vi "Microscope Controller GFV.vi"(8 "error in (no error)":errorcluster, 10 "MicroscopeEnum":T1, 11 "Data in":variant) -> (0 "error out":errorcluster, 3 "Data Out":variant)   [LabVIEW 2017]
doc: "Use this template to build a VI to use as a subVI."
uses:
  Microscope/MicroscopeControllerEnum.ctl
  Microscope/MicroscopeControllerCluster.ctl
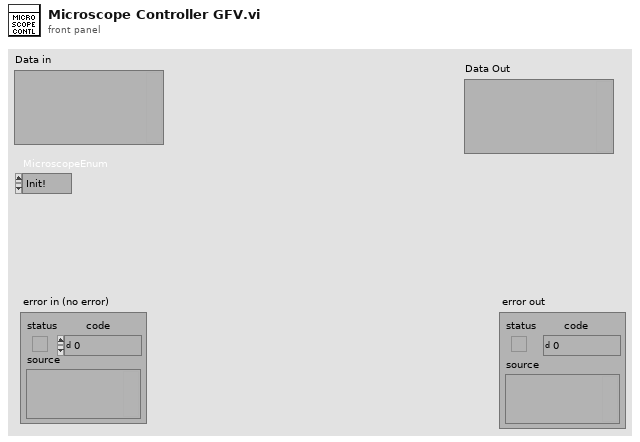
[diagram p1: front panel]
types:
  T1 = typedef "MicroscopeControllerEnum.ctl" = enum16{"Init!", "Start!", "Stop!", "GetMicroscopeVIRef", "InsertCallbackEvent!"}
  T2 = typedef "MicroscopeControllerCluster.ctl" = cluster{"MapPointsArray":cluster{"X":i32, "Y":i32}[], "Laser Point Coor":cluster{"X":i32, "Y":i32}, "Microscope \nObjective":u16}
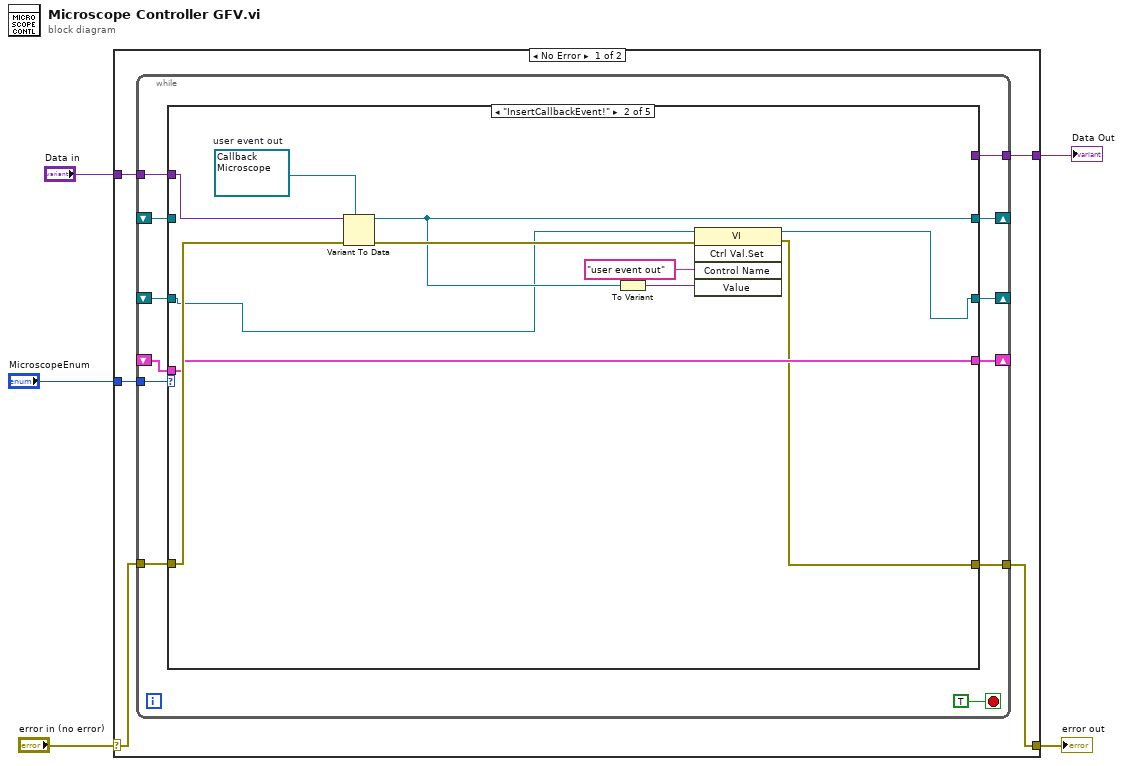
[diagram p0: block diagram]
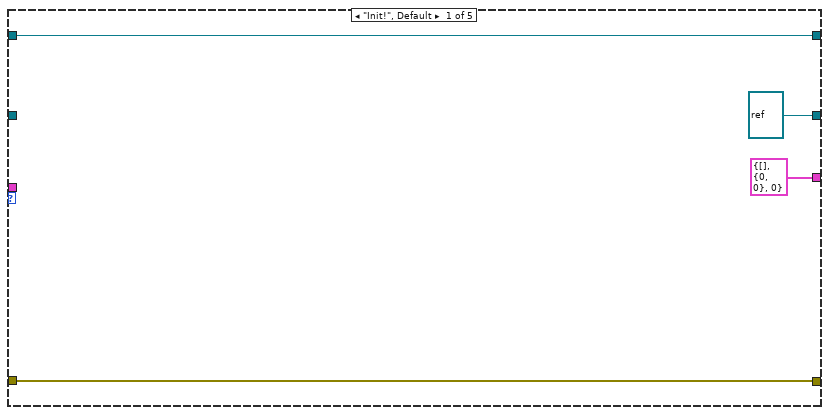
[diagram p2: hidden frame]
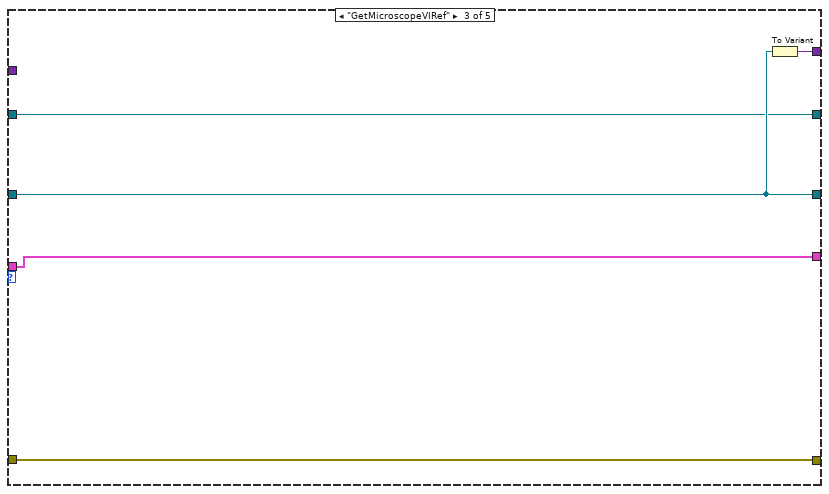
[diagram p3: hidden frame]
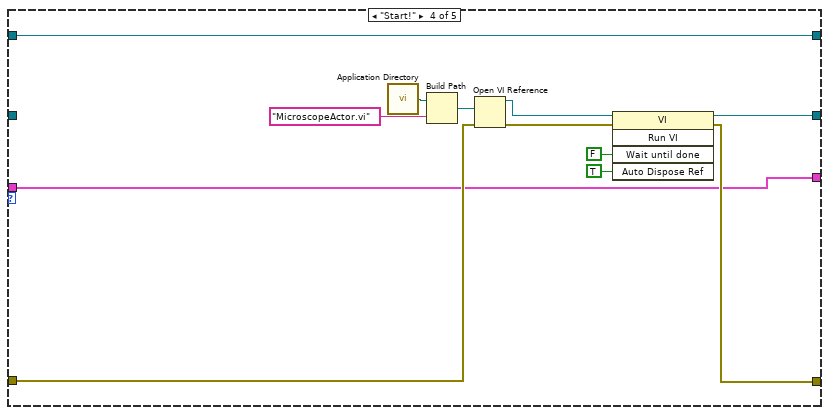
[diagram p4: hidden frame]
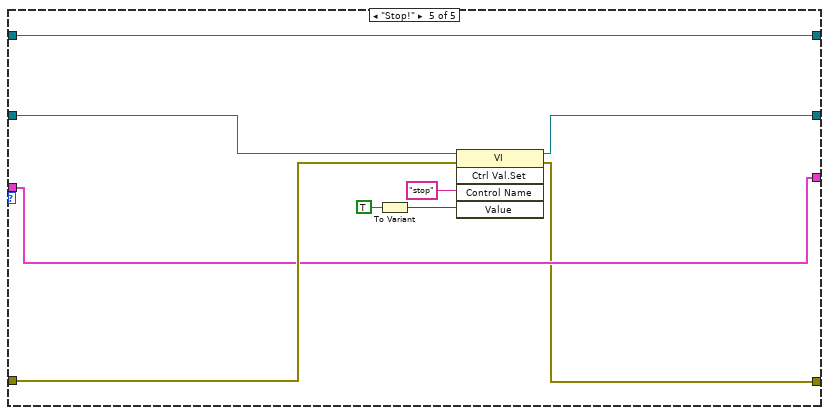
[diagram p5: hidden frame]
diagram:
  n1 = case shown="No Error" "error in (no error)" {
    selector: "error in (no error)" -> [w9 w64]
    tunnel: [w8 w64] -> w4
    tunnel: "MicroscopeEnum" -> [w10 _]
    tunnel: [w7 _] -> w2
    tunnel: "Data in" -> [w6 _]
    frame No Error {
      n2 = while {
        tunnel: w10 -> [w21]
        tunnel: w9 -> [w20]
        shift-right: [w18] -> _
        shift-left: _ -> [w16]
        shift-right: [w19] -> _
        shift-left: _ -> [w15]
        tunnel: [w17] -> w8
        tunnel: [w14] -> w7
        shift-right: [w12] -> _
        shift-left: _ -> [w13]
        tunnel: w6 -> [w11]
        stop <- TRUE stop-if-true
        n3 = case shown="\"InsertCallbackEvent!\"" w21 {
          tunnel: w20 -> [w24 w33 w41 w47 w60]
          tunnel: [refnum<vi> refnum ("vi reference") w30 w40 w45 w58] -> w19
          tunnel: [T2 {"MapPointsArray"=[], "Laser Point Coor"={"X"=0, "Y"=0}, "Microscope \nObjective"=0} w32 w42 w44 w57] -> w18
          tunnel: [w24 w28 w41 w46 w56] -> w17
          tunnel: w16 -> [_ w32 w42 w44 w57]
          tunnel: w15 -> [_ w31 w40 _ w59]
          tunnel: [_ _ w39 _ _] -> w14
          tunnel: w13 -> [w23 _ w38 w43 w55]
          tunnel: [w23 w34 w38 w43 w55] -> w12
          tunnel: w11 -> [_ w29 _ _ _]
          frame "Init!", Default {
          }
          frame "InsertCallbackEvent!" {
            w27 = refnum<user-event> refnum  # user event out
            n4 = Variant To Data(error in=w33, type=w27, Variant=w29) -> (data=w34:refnum<user-event>, error out=w35:errorcluster)
            n5 = To Variant(anything=w34) -> (Variant=w37:variant)
            n6 = invoke class="VI" method="Ctrl Val.Set"(reference=w31, error in=w35, "Control Name"="user event out", "Value"=w37) -> (reference out=w30:refnum<vi>, error out=w28:errorcluster)  [unwired: 1 in, 3 out]
          }
          frame "GetMicroscopeVIRef" {
            n7 = To Variant(anything=w40) -> (Variant=w39:variant)
          }
          frame "Start!" {
            n8 = call <vilib>:"Application Directory.vi"() -> ("Application Directory"=w52:path)
            n9 = Build Path(base path=w52, name or relative path="MicroscopeActor.vi") -> (appended path=w50:path)
            n10 = Open VI Reference(vi path=w50, error in (no error)=w47) -> (vi reference=w48:refnum<vi>, error out=w49:errorcluster)  [unwired: 4 in]
            n11 = invoke class="VI" method="Run VI"(reference=w48, error in=w49, "Wait until done"=FALSE ("Wait Until Done"), "Auto Dispose Ref"=TRUE ("Auto Dispose Reference")) -> (reference out=w45:refnum<vi>, error out=w46:errorcluster)  [unwired: 1 in, 3 out]
          }
          frame "Stop!" {
            n12 = To Variant(anything=TRUE) -> (Variant=w62:variant)
            n13 = invoke class="VI" method="Ctrl Val.Set"(reference=w59, error in=w60, "Control Name"="stop", "Value"=w62) -> (reference out=w58:refnum<vi>, error out=w56:errorcluster)  [unwired: 1 in, 3 out]
          }
        }
      }
    }
    frame Error {
    }
  }
  "error out" <- w4
  "Data Out" <- w2
